vi "Finish.vi"   [LabVIEW 2017]
doc: "This VI is called just before exiting. It is expected to close I/O refnum, save collected data, etc."
uses:
  <vilib>/Rock Robotics/WPI/Utilities/WPI_GetSetVariantRefNum.vi
types:
  T1 = typedef "WPI_MotorControlDeviceRef.ctl" = cluster{"DeviceStatus":errorcluster, "Type":T2, "PWM":cluster{"PWM Channel":T3, "DeadBand":T4}, "CAN":cluster{"Device Number":u8, "SetOutput VI Ref":variant, "GetOutput VI Ref":variant, "Enable VI Ref":variant, "Disable VI Ref":variant, "Data":variant}, "Invert":bool, "DIO PWM":cluster{"PWM \"Enable\" Channel":T3, "DIOChannel":T5, "PWM Rate":dbl}}
  T2 = typedef "WPI_MotorControlType.ctl" = enum16{"PWM", "CAN", "DIO PWM"}
  T3 = typedef "FPGA_DIOPWMChannel.ctl" = enum8{"PWM 0", "PWM 1", "PWM 2", "PWM 3", "PWM 4", "PWM 5", "PWM 6", "PWM 7", "PWM 8", "PWM 9", "PWM MXP 0", "PWM MXP 1", "PWM MXP 2", "PWM MXP 3", "PWM MXP 4", "PWM MXP 5", "PWM MXP 6", "PWM MXP 7", "PWM MXP 8", "PWM MXP 9", "Invalid"}
  T4 = typedef "WPI_PWMDeadband.ctl" = cluster{"Name":string, "maxPositivePwm":i32, "minPositivePwm":i32, "centerPwm":i32, "maxNegativePwm":i32, "minNegativePwm":i32, "angularRange":u16}
  T5 = typedef "FPGA_DIOChannel.ctl" = enum8{"DIO 0", "DIO 1", "DIO 2", "DIO 3", "DIO 4", "DIO 5", "DIO 6", "DIO 7", "DIO 8", "DIO 9", "DIO MXP 0", "DIO MXP 1", "DIO MXP 2", "DIO MXP 3", "DIO MXP 4", "DIO MXP 5", "DIO MXP 6", "DIO MXP 7", "DIO MXP 8", "DIO MXP 9", "DIO MXP 10", "DIO MXP 11", "DIO MXP 12", "DIO MXP 13", "DIO MXP 14", "DIO MXP 15", "SPI Port CS1", "SPI Port CS2", "SPI Port CS3", "SPI Port MISO", "SPI Port MOSI", "Invalid"}
  T6 = typedef "WPI_JoystickDevRef.ctl" = cluster{"Device":T7}
  T7 = typedef "WPI_JoystickDeviceEnum.ctl" = enum16{"USB 0", "USB 1", "USB 2", "USB 3", "USB 4", "USB 5"}
  T8 = typedef "WPI_SolenoidDevRef.ctl" = cluster{"DevStatus":errorcluster, "Pneumatics Control Module":u8, "Forward Solenoid Channel":T9, "Reverse Solenoid Channel":T9}
  T9 = typedef "WPI_SolenoidChannel.ctl" = enum8{"Solenoid 0", "Solenoid 1", "Solenoid 2", "Solenoid 3", "Solenoid 4", "Solenoid 5", "Solenoid 6", "Solenoid 7", "Invalid"}
  T10 = typedef "WPI_ServoDeviceRef.ctl" = cluster{"DeviceStatus":errorcluster, "PWM Channel":T3, "DeadBand":T4}
  T11 = typedef "WPI_SwitchDevRef.ctl" = cluster{"DevStatus":errorcluster, "DIO Channel":T5, "CntIndex":T12, "Normally Closed":bool}
  T12 = typedef "FPGA_CounterCtrSystemIndex.ctl" = enum8{"Ctr 0", "Ctr 1", "Ctr 2", "Ctr 3", "Ctr 4", "Ctr 5", "Ctr 6", "Ctr 7", "Invalid"}
  T13 = typedef "WPI_EncoderDevRef.ctl" = cluster{"DevStatus":errorcluster, "EncoderIndex":T14, "CounterIndex":T12, "DistancePerCount":dbl, "Decoding Type":T15}
  T14 = typedef "FPGA_EncoderIdx.ctl" = enum8{"Enc 0", "Enc 1", "Enc 2", "Enc 3", "Enc 4", "Enc 5", "Enc 6", "Enc 7", "Invalid"}
  T15 = typedef "WPI_EncoderType.ctl" = enum16{"1x", "2x", "4x"}
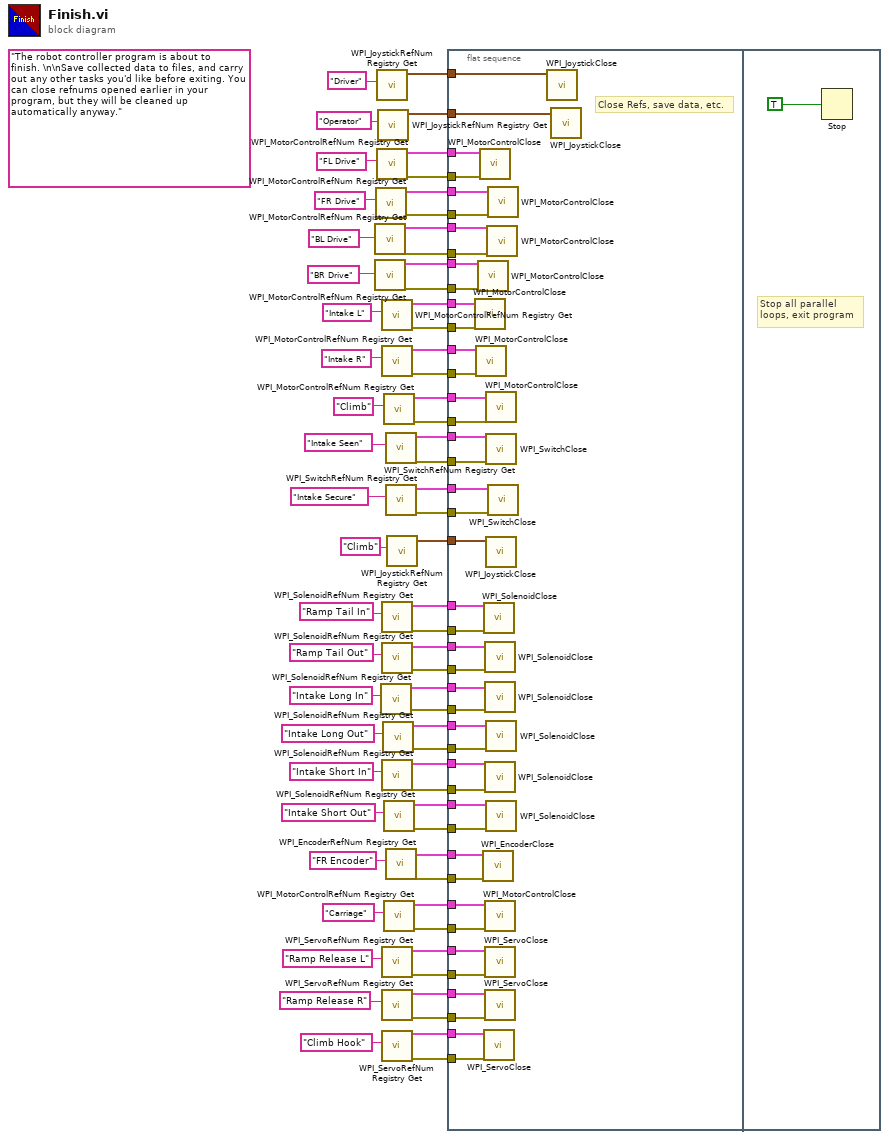
[diagram p0: block diagram]
diagram:
  (unwired) "The robot controller program is about to finish. \n\nSave collected data to files, and carry out any other tasks you'd like before exiting. You can close refnums opened earlier in your program, but they will be cleaned up automatically anyway."
  n1 = call <vilib>:"WPI_MotorControlRefNum Registry Get.vi"("refnum name"="BL Drive") -> ("error out"=w23:errorcluster, "MotorControlDevRef"=w24:T1)  [unwired: 9 in]
  n2 = call <vilib>:"WPI_MotorControlRefNum Registry Get.vi"("refnum name"="BR Drive") -> ("error out"=w21:errorcluster, "MotorControlDevRef"=w22:T1)  [unwired: 9 in]
  n3 = call <vilib>:"WPI_MotorControlRefNum Registry Get.vi"("refnum name"="FR Drive") -> ("error out"=w25:errorcluster, "MotorControlDevRef"=w26:T1)  [unwired: 9 in]
  n4 = call <vilib>:"WPI_JoystickRefNum Registry Get.vi"("refnum name"="Driver") -> ("JoystickDevRef"=w65:T6)  [unwired: 1 in, 9 out]
  n5 = call <vilib>:"WPI_MotorControlRefNum Registry Get.vi"("refnum name"="FL Drive") -> ("error out"=w27:errorcluster, "MotorControlDevRef"=w28:T1)  [unwired: 9 in]
  n6 = call <vilib>:"WPI_JoystickRefNum Registry Get.vi"("refnum name"="Operator") -> ("JoystickDevRef"=w63:T6)  [unwired: 1 in, 9 out]
  n7 = call <vilib>:"WPI_SolenoidRefNum Registry Get.vi"("refnum name"="Intake Long In") -> ("error out"=w39:errorcluster, "SolenoidDevRef"=w40:T8)  [unwired: 9 in]
  n8 = call <vilib>:"WPI_MotorControlRefNum Registry Get.vi"("refnum name"="Intake L") -> ("error out"=w58:errorcluster, "MotorControlDevRef"=w60:T1)  [unwired: 9 in]
  n9 = call <vilib>:"WPI_MotorControlRefNum Registry Get.vi"("refnum name"="Intake R") -> ("error out"=w1:errorcluster, "MotorControlDevRef"=w2:T1)  [unwired: 9 in]
  n10 = call <vilib>:"WPI_SolenoidRefNum Registry Get.vi"("refnum name"="Ramp Tail In") -> ("error out"=w43:errorcluster, "SolenoidDevRef"=w44:T8)  [unwired: 9 in]
  n11 = call <vilib>:"WPI_SolenoidRefNum Registry Get.vi"("refnum name"="Ramp Tail Out") -> ("error out"=w41:errorcluster, "SolenoidDevRef"=w42:T8)  [unwired: 9 in]
  n12 = call <vilib>:"WPI_SolenoidRefNum Registry Get.vi"("refnum name"="Intake Short In") -> ("error out"=w35:errorcluster, "SolenoidDevRef"=w36:T8)  [unwired: 9 in]
  n13 = call <vilib>:"WPI_ServoRefNum Registry Get.vi"("refnum name"="Ramp Release L") -> ("error out"=w12:errorcluster, "ServoDeviceRef"=w11:T10)  [unwired: 9 in]
  n14 = call <vilib>:"WPI_ServoRefNum Registry Get.vi"("refnum name"="Ramp Release R") -> ("error out"=w13:errorcluster, "ServoDeviceRef"=w14:T10)  [unwired: 9 in]
  n15 = call <vilib>:"WPI_ServoRefNum Registry Get.vi"("refnum name"="Climb Hook") -> ("error out"=w6:errorcluster, "ServoDeviceRef"=w7:T10)  [unwired: 9 in]
  n16 = call <vilib>:"WPI_SolenoidRefNum Registry Get.vi"("refnum name"="Intake Long Out") -> ("error out"=w37:errorcluster, "SolenoidDevRef"=w38:T8)  [unwired: 9 in]
  n17 = call <vilib>:"WPI_MotorControlRefNum Registry Get.vi"("refnum name"="Climb") -> ("error out"=w57:errorcluster, "MotorControlDevRef"=w59:T1)  [unwired: 9 in]
  n18 = call <vilib>:"WPI_SolenoidRefNum Registry Get.vi"("refnum name"="Intake Short Out") -> ("error out"=w33:errorcluster, "SolenoidDevRef"=w34:T8)  [unwired: 9 in]
  n19 = call <vilib>:"WPI_MotorControlRefNum Registry Get.vi"("refnum name"="Carriage") -> ("error out"=w16:errorcluster, "MotorControlDevRef"=w17:T1)  [unwired: 9 in]
  n20 = call <vilib>:"WPI_SwitchRefNum Registry Get.vi"("refnum name"="Intake Seen") -> ("error out"=w54:errorcluster, "SwitchDevRef"=w55:T11)  [unwired: 9 in]
  n21 = call <vilib>:"WPI_SwitchRefNum Registry Get.vi"("refnum name"="Intake Secure") -> ("error out"=w53:errorcluster, "SwitchDevRef"=w56:T11)  [unwired: 9 in]
  n22 = call <vilib>:"WPI_EncoderRefNum Registry Get.vi"("refnum name"="FR Encoder") -> ("error out"=w18:errorcluster, "EncoderDevRef"=w19:T13)  [unwired: 9 in]
  n23 = call <vilib>:"WPI_JoystickRefNum Registry Get.vi"("refnum name"="Climb") -> ("JoystickDevRef"=w4:T6)  [unwired: 1 in, 9 out]
  n24 = flat-sequence {
    tunnel: w65 -> [w109]
    tunnel: w63 -> [w108]
    tunnel: w60 -> [w107]
    tunnel: w59 -> [w106]
    tunnel: w58 -> [w105]
    tunnel: w57 -> [w104]
    tunnel: w56 -> [w103]
    tunnel: w55 -> [w102]
    tunnel: w54 -> [w101]
    tunnel: w53 -> [w100]
    tunnel: w44 -> [w99]
    tunnel: w43 -> [w98]
    tunnel: w42 -> [w97]
    tunnel: w41 -> [w96]
    tunnel: w40 -> [w95]
    tunnel: w39 -> [w94]
    tunnel: w38 -> [w93]
    tunnel: w37 -> [w92]
    tunnel: w36 -> [w91]
    tunnel: w35 -> [w90]
    tunnel: w34 -> [w89]
    tunnel: w33 -> [w88]
    tunnel: w28 -> [w87]
    tunnel: w27 -> [w86]
    tunnel: w26 -> [w85]
    tunnel: w25 -> [w84]
    tunnel: w24 -> [w83]
    tunnel: w23 -> [w82]
    tunnel: w22 -> [w81]
    tunnel: w21 -> [w80]
    tunnel: w19 -> [w79]
    tunnel: w18 -> [w78]
    tunnel: w17 -> [w76]
    tunnel: w16 -> [w77]
    tunnel: w14 -> [w75]
    tunnel: w13 -> [w74]
    tunnel: w12 -> [w73]
    tunnel: w11 -> [w72]
    tunnel: w7 -> [w71]
    tunnel: w6 -> [w70]
    tunnel: w4 -> [w69]
    tunnel: w2 -> [w68]
    tunnel: w1 -> [w67]
    frame #0 {
      # "Close Refs, save data, etc."
      n25 = call <vilib>:"WPI_MotorControlClose.vi"("error in"=w105, "MotorControlDevRef"=w107) -> ()  [unwired: 9 in, 1 out]
      n26 = call <vilib>:"WPI_MotorControlClose.vi"("error in"=w67, "MotorControlDevRef"=w68) -> ()  [unwired: 9 in, 1 out]
      n27 = call <vilib>:"WPI_MotorControlClose.vi"("error in"=w80, "MotorControlDevRef"=w81) -> ()  [unwired: 9 in, 1 out]
      n28 = call <vilib>:"WPI_MotorControlClose.vi"("error in"=w86, "MotorControlDevRef"=w87) -> ()  [unwired: 9 in, 1 out]
      n29 = call <vilib>:"WPI_EncoderClose.vi"("error in (no error)"=w78, "EncoderDevRef"=w79) -> ()  [unwired: 9 in, 1 out]
      n30 = call <vilib>:"WPI_SolenoidClose.vi"("error in (no error)"=w98, "SolenoidDevRef"=w99) -> ()  [unwired: 9 in, 1 out]
      n31 = call <vilib>:"WPI_ServoClose.vi"("error in (no error)"=w70, "ServoDeviceRef"=w71) -> ()  [unwired: 9 in, 1 out]
      n32 = call <vilib>:"WPI_SolenoidClose.vi"("error in (no error)"=w96, "SolenoidDevRef"=w97) -> ()  [unwired: 9 in, 1 out]
      n33 = call <vilib>:"WPI_SolenoidClose.vi"("error in (no error)"=w94, "SolenoidDevRef"=w95) -> ()  [unwired: 9 in, 1 out]
      n34 = call <vilib>:"WPI_SolenoidClose.vi"("error in (no error)"=w90, "SolenoidDevRef"=w91) -> ()  [unwired: 9 in, 1 out]
      n35 = call <vilib>:"WPI_MotorControlClose.vi"("error in"=w77, "MotorControlDevRef"=w76) -> ()  [unwired: 9 in, 1 out]
      n36 = call <vilib>:"WPI_ServoClose.vi"("error in (no error)"=w73, "ServoDeviceRef"=w72) -> ()  [unwired: 9 in, 1 out]
      n37 = call <vilib>:"WPI_ServoClose.vi"("error in (no error)"=w74, "ServoDeviceRef"=w75) -> ()  [unwired: 9 in, 1 out]
      n38 = call <vilib>:"WPI_MotorControlClose.vi"("error in"=w104, "MotorControlDevRef"=w106) -> ()  [unwired: 9 in, 1 out]
      n39 = call <vilib>:"WPI_SwitchClose.vi"("error in (no error)"=w101, "SwitchDevRef"=w102) -> ()  [unwired: 9 in, 1 out]
      n40 = call <vilib>:"WPI_JoystickClose.vi"("JoystickDevRef"=w69) -> ()  [unwired: 11 out]
      n41 = call <vilib>:"WPI_SolenoidClose.vi"("error in (no error)"=w92, "SolenoidDevRef"=w93) -> ()  [unwired: 9 in, 1 out]
      n42 = call <vilib>:"WPI_SolenoidClose.vi"("error in (no error)"=w88, "SolenoidDevRef"=w89) -> ()  [unwired: 9 in, 1 out]
      n43 = call <vilib>:"WPI_MotorControlClose.vi"("error in"=w82, "MotorControlDevRef"=w83) -> ()  [unwired: 9 in, 1 out]
      n44 = call <vilib>:"WPI_MotorControlClose.vi"("error in"=w84, "MotorControlDevRef"=w85) -> ()  [unwired: 9 in, 1 out]
      n45 = call <vilib>:"WPI_SwitchClose.vi"("error in (no error)"=w100, "SwitchDevRef"=w103) -> ()  [unwired: 9 in, 1 out]
      n46 = call <vilib>:"WPI_JoystickClose.vi"("JoystickDevRef"=w109) -> ()  [unwired: 11 out]
      n47 = call <vilib>:"WPI_JoystickClose.vi"("JoystickDevRef"=w108) -> ()  [unwired: 11 out]
    }
    frame #1 {
      # "Stop all parallel\nloops, exit program"
      n48 = Stop(stop? (T)=TRUE ("Quit")) -> ()
    }
  }
